vi "QMH UI.vi"() -> ()   [LabVIEW 2026]
panel:
  in  "stop":bool
  in  "iperfTest":bool
  in  "LOG":bool
  in  "PING":bool
  out "DASHBOARD":string[][](table)
  in  "SETTINGS":T1(tab)
  in  "XNET INTERFACE":u32(ring) items=["ENET1", "ENET2"]
  in  "PORT CONFIGURATION":T2(array[cluster])
  in  "SPEED":u32(ring) items=["1000Mb/s", "100Mb/s"]
  in  "SLEEP CAPABILITY":u32(ring) items=["Disabled", "Enabled"]
  in  "PROTOCOL":string(combo)
  in  "DIRECTION":string(combo)
  in  "LISTEN PORT":u16
  in  "DUT iPERF TEST PORT":u16
  in  "DUT SSH PORT":u16
  in  "DUT Password":string
  in  "DUT Username":string="Administrator"
  in  "DUT IP":string="192.168.1.3"
  in  "DURATION iPERF TEST (s)":u16
  in  "Force traffic (UDP only)":T3(ring)
  in  "Protocol":enum16{"UDP", "TCP"}(ring)=enum."TCP"
  in  "CLIENT iPERF PORT":u16
  in  "CONTINUOUS TEST":bool=TRUE
  out "Ping":bool
  out "Server results":T4
  out "Client results":T4
  out "Link Status":T5
  in  "PuTTY root folder":path=path "C:/DEV/emea-tra-iPerf_bus_load_test/utility/Putty_ssh_client"
  in  "iPerf_path_remote_client":path=path "C:/DEV/emea-tra-iPerf_bus_load_test/utility/iperf3.17.1_64" caption="iPerf root folder CLIENT"
  in  "iPerf_path_remote_server":path=path "C:/DEV/emea-tra-iPerf_bus_load_test/utility/iperf3.17.1_64" caption="iPerf root folder SERVER"
  in  "Stack mode":enum16{"OS stack", "IP stack"}(ring)
  # "CONFIGURATION"
  # "RESULTS"
  # "Tests"
  # "STATUS"
  # "CONTROL"
  # "TODO: Need to format these settings once defined which one we'll need"
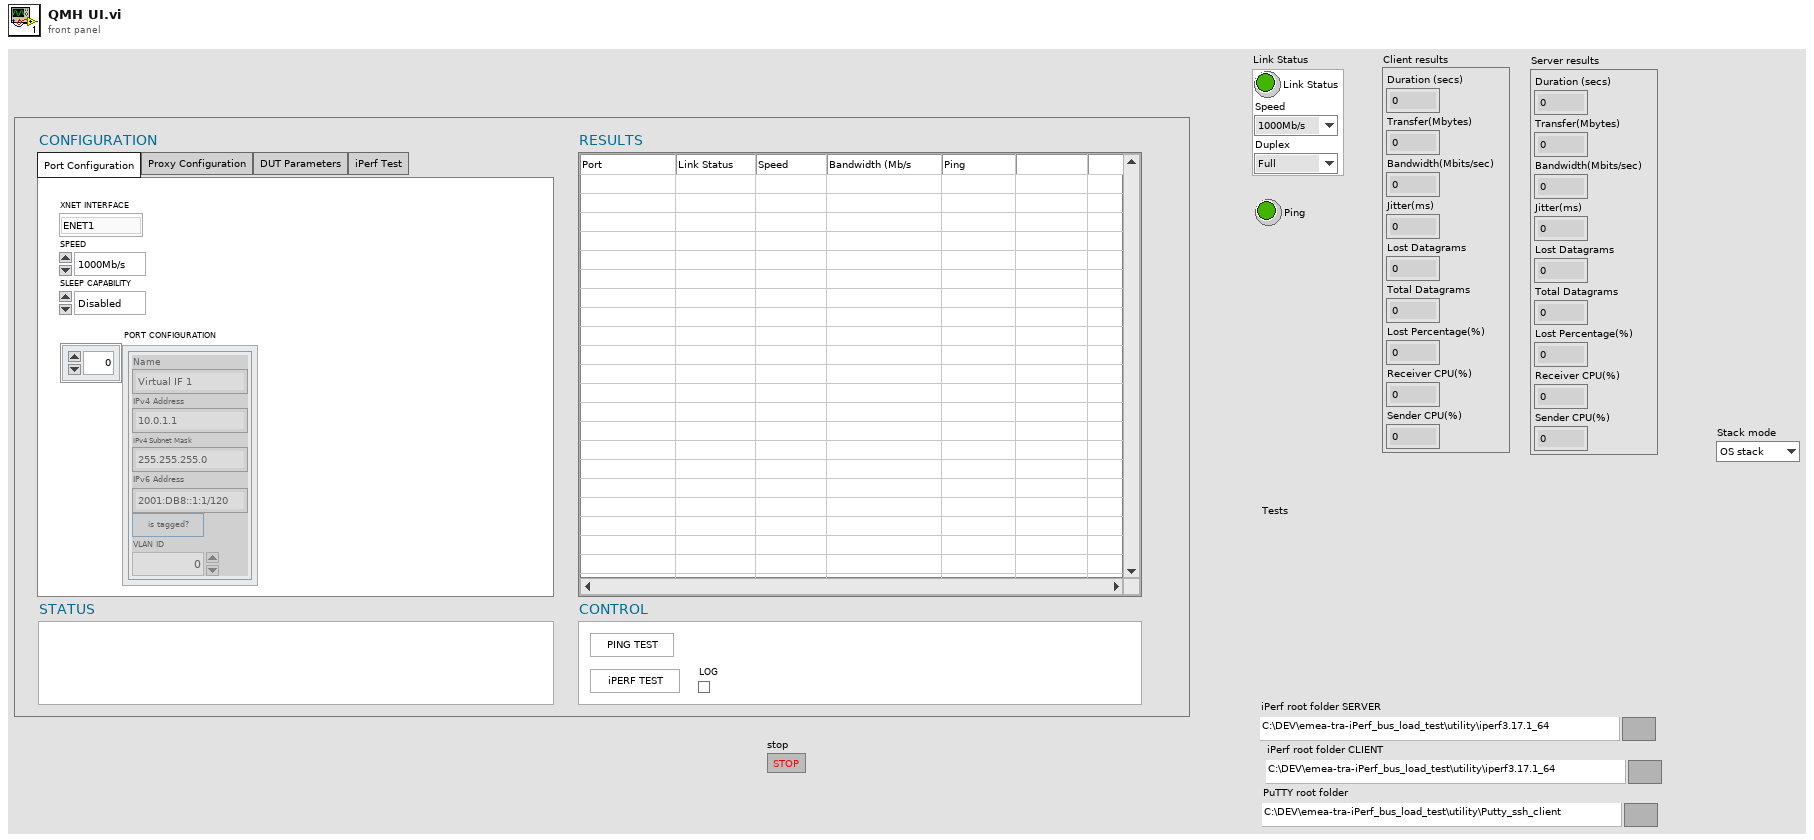
[diagram p1: front panel]
types:
  T1 = enum32{"Port Configuration", "Proxy Configuration", "DUT Parameters", "iPerf Test"}
  T2 = cluster{"Name":string, "IPv4 Address":string, "IPv4 Subnet Mask":string, "IPv6 Address":string, "is tagged?":bool, "VLAN ID":u16}[]
  T3 = enum16{"1M", "10M", "20M", "30M", "40M", "50M", "100M", "500M", "1000M"}
  T4 = cluster{"Duration (secs)":dbl, "Transfer(Mbytes)":dbl, "Bandwidth(Mbits/sec)":dbl, "Jitter(ms)":dbl, "Lost Datagrams":i32, "Total Datagrams":i32, "Lost Percentage(%)":dbl, "Receiver CPU(%)":dbl, "Sender CPU(%)":dbl}
  T5 = cluster{"Link Status":bool, "Speed":enum16{"1000Mb/s", "100Mb/s"}, "Duplex":enum16{"Full", "Half"}}
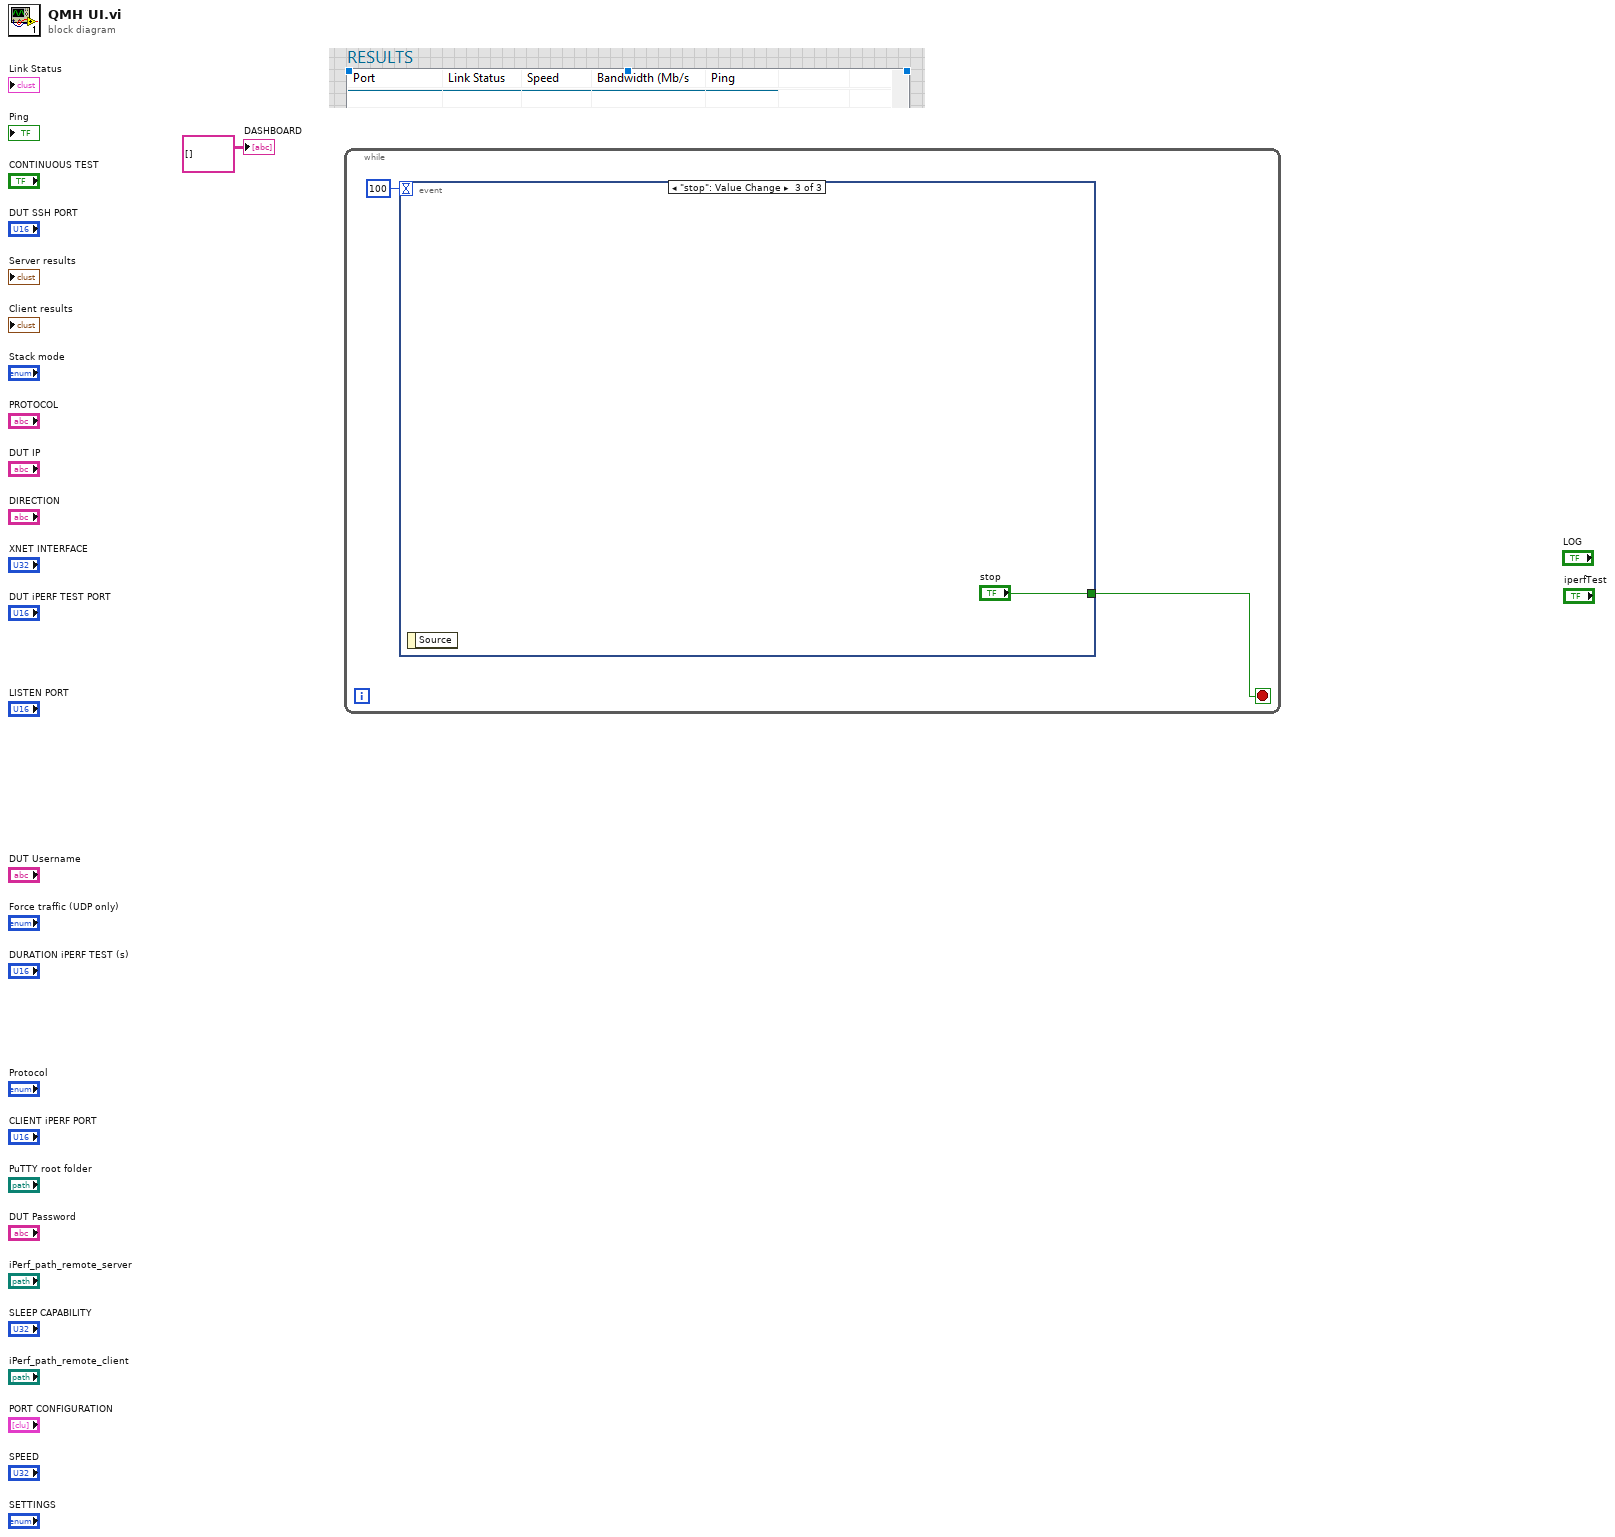
[diagram p0: block diagram]
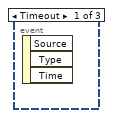
[diagram p2: hidden frame]
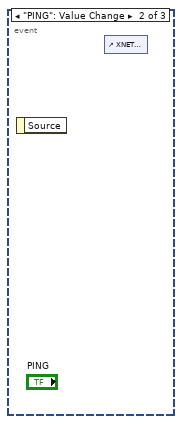
[diagram p3: hidden frame]
diagram:
  n1 = while {
    stop <- w2 stop-if-true
    n2 = event shown="[2] \"stop\": Value Change" {
      selector: _ -> [_ _ _]
      dyn-events: _ -> [_ _ _]
      timeout: 100 -> [_ _ _]
      tunnel: [_ _ "stop"] -> w2
      event Timeout {
        n3 = event-data() -> ()  [unwired: 1 in, 3 out]
      }
      event "PING": Value Change {
        n4 = event-data() -> ()  [unwired: 1 in, 1 out]
        n5 = control-ref of="XNET INTERFACE"() -> ()  [unwired: 1 out]
      }
      event "stop": Value Change {
        n6 = event-data() -> ()  [unwired: 1 in, 1 out]
      }
    }
  }
  "DASHBOARD" <- string[][] [] ("DASHBOARD")
